vi "Write ILCADC.vi"(10 "ADC Collection Settings":T1={"Input Channels"=enum."Channel 0", "Scan Rate (Hz) "=enum."4800", "PGA Gain Coefficient"=0} {"PGA Gain Coefficient" max=7}, 11 "ILCSim1 in":refnum<class "ILCSim1.lvclass">) -> (3 "ILCSim1 out":refnum<class "ILCSim1.lvclass">)   [LabVIEW 2015, in "ILCSim1.lvclass"]
uses:
  <userlib>/Common/Simulators/ILCSim1/ILCSim1.lvclass
  <userlib>/Common/ILC/Configuration/ADC Collection Settings.ctl
  <userlib>/Common/ILC/Configuration/Input Channels.ctl
  <userlib>/Common/ILC/Configuration/Scan Rates.ctl
  <userlib>/Common/Simulators/ILCSim1/ILCSim1.lvclass/ILCSim1.ctl
  <userlib>/Common/ILC/Configuration/ILCConfiguration.lvlib
panel:
  # "Gain is 2^gain_coefficient"
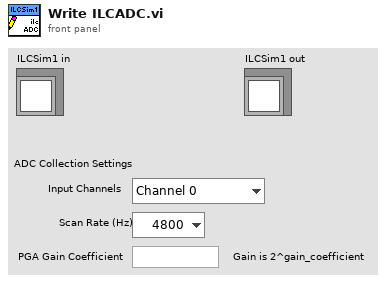
[diagram p1: front panel]
types:
  T1 = typedef "ILCCommon.lvlib/ILCConfiguration.lvlib/ADC Collection Settings.ctl" = cluster{"Input Channels":T2, "Scan Rate (Hz) ":T3, "PGA Gain Coefficient":u8}
  T2 = typedef "ILCCommon.lvlib/ILCConfiguration.lvlib/Input Channels.ctl" = enum16{"Channel 0", "3 Channels", "5 Channels"}
  T3 = typedef "ILCCommon.lvlib/ILCConfiguration.lvlib/Scan Rates.ctl" = enum16{"50", "60", "100", "120", "200", "240", "300", "400", "480", "600", "1200", "2400", "4800"}
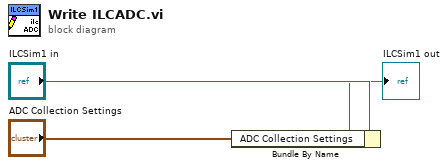
[diagram p0: block diagram]
diagram:
  n1 = Bundle By Name(cluster="ILCSim1 in", "ADC Collection Settings"="ADC Collection Settings") -> (→"ILCSim1 out":refnum<class "ILCSim1.lvclass">)
